vi "Identify Trigger Hysteresis.vi"(7 "Start Trigger Refnum":refnum<vi>, 8 "Error in":errorcluster, 10 "Detection Result":bool, 11 "State Variables in":T1={"Stop Notifier"=refnum, "UI References"=[], "DAQmx"={"ECG Input"={"Channel"="", "Task"="", "Max Value"=0.0, "Min Value"=0.0, "Sampling Rate"=0.0, "Batch Size"=10}, "Trigger Output"={"Channel"="", "Task"="", "Pulse Frequency"=0.0, "Delay"=0, "Triggers per Shot"=0}}, "Data Queue"=refnum, "Filter"={"Batch Size"=1000, "Update Cycle"=0, "Filter Buffer"=[]}, "Last Detect Result"=FALSE}) -> (0 "Error out":errorcluster, 2 "Hysteresis Trigger":bool, 3 "State Variables out":T1={"Stop Notifier"=refnum, "UI References"=[], "DAQmx"={"ECG Input"={"Channel"="", "Task"="", "Max Value"=0.0, "Min Value"=0.0, "Sampling Rate"=0.0, "Batch Size"=10}, "Trigger Output"={"Channel"="", "Task"="", "Pulse Frequency"=0.0, "Delay"=0, "Triggers per Shot"=0}}, "Data Queue"=refnum, "Filter"={"Batch Size"=1000, "Update Cycle"=0, "Filter Buffer"=[]}, "Last Detect Result"=FALSE})   [LabVIEW 2014, in "Trigger Output.lvlib"]
uses:
  Trigger Output.lvlib
  Controls/State Variables.ctl
  Controls/DAQmx Variables.ctl
  Controls/Filter Variables.ctl
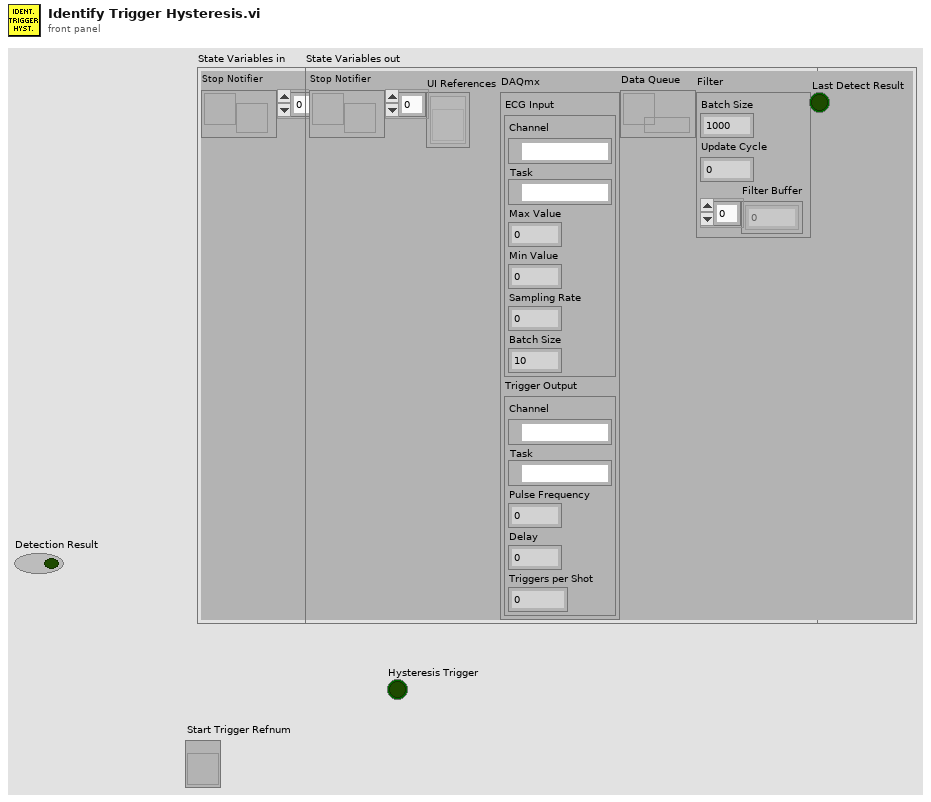
[diagram p1: front panel]
types:
  T1 = typedef "State Variables.ctl" = cluster{"Stop Notifier":refnum<notifier>, "UI References":refnum<vi>[], "DAQmx":T2, "Data Queue":refnum<queue>, "Filter":T3, "Last Detect Result":bool}
  T2 = typedef "DAQmx Variables.ctl" = cluster{"ECG Input":cluster{"Channel":tag, "Task":refnum<k21>, "Max Value":dbl, "Min Value":dbl, "Sampling Rate":dbl, "Batch Size":i32}, "Trigger Output":cluster{"Channel":tag, "Task":refnum<k21>, "Pulse Frequency":dbl, "Delay":u16, "Triggers per Shot":i32}}
  T3 = typedef "Filter Variables.ctl" = cluster{"Batch Size":i32, "Update Cycle":i32, "Filter Buffer":dbl[]}
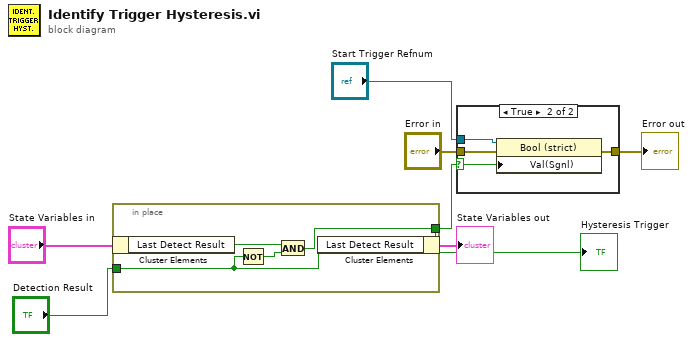
[diagram p0: block diagram]
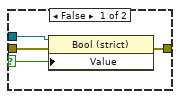
[diagram p2: hidden frame]
diagram:
  n1 = in-place {
    in-place-border: "Detection Result" -> [w9]
    in-place-border: [w8] -> w4
    n2 = in-place-cluster #1("State Variables in") -> ("Last Detect Result"=w11:bool)
    n3 = Not(x=w9) -> (.not. x?=w10:bool)
    n4 = And(x=w11, y=w10) -> (x .and. y?=w8:bool)
    n5 = in-place-cluster #1("Last Detect Result"=w9) -> (→"State Variables out":T1)
  }
  "Hysteresis Trigger" <- w4
  n6 = case shown="True" w4 {
    selector: w4 -> [w15 w16]
    tunnel: "Error in" -> [w14 w19]
    tunnel: [w12 w18] -> w2
    tunnel: "Start Trigger Refnum" -> [w13 w17]
    frame False {
      n7 = property class="Bool (strict)"(reference=w13, error in=w14, "Value"=w15) -> (error out=w12:errorcluster)  [unwired: 1 out]
    }
    frame True {
      n8 = property class="Bool (strict)"(reference=w17, error in=w19, "Val(Sgnl)"=w16) -> (error out=w18:errorcluster)  [unwired: 1 out]
    }
  }
  "Error out" <- w2
